vi "TwoSensorMagazineLogic.vi"(0 "Intake Toggle":bool, 1 "Outtake Button":bool, 2 "error in (no error)":errorcluster, 3 "Outtake Side Sensor":bool, 4 "Intake Side Sensor":bool) -> (5 "Current State":T1, 6 "Intake Pistons":bool, 7 "Magazine Motors":dbl, 8 "Kicker Motors":dbl, 9 "Intake Motors":dbl, 10 "error out":errorcluster)   [LabVIEW 2020]
uses:
  MagazineControl.ctl
  TitanLib/Lib/TitanLib.lvlib
panel:
  in  "Kicker Power":dbl=0.5
  in  "Magazine Power":dbl=1.0
  in  "Input Power":dbl=1.0
  in  "Initial State":T1
  # "Inputs"
  # "Power Levels"
  # "Outputs"
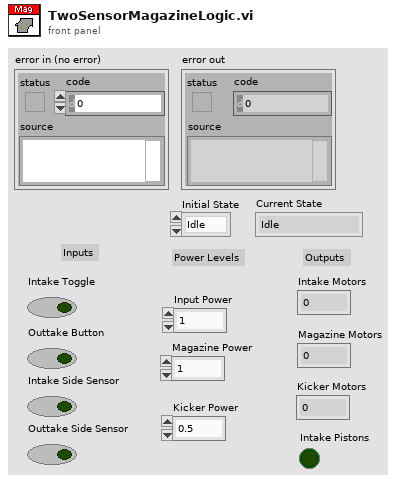
[diagram p1: front panel]
types:
  T1 = typedef "MagazineControl.ctl" = enum16{"Idle", "Intaking", "Outtake", "One Ball", "One Ball Intake", "One Ball Outtake", "Two Balls", "Two Ball Outtake"}
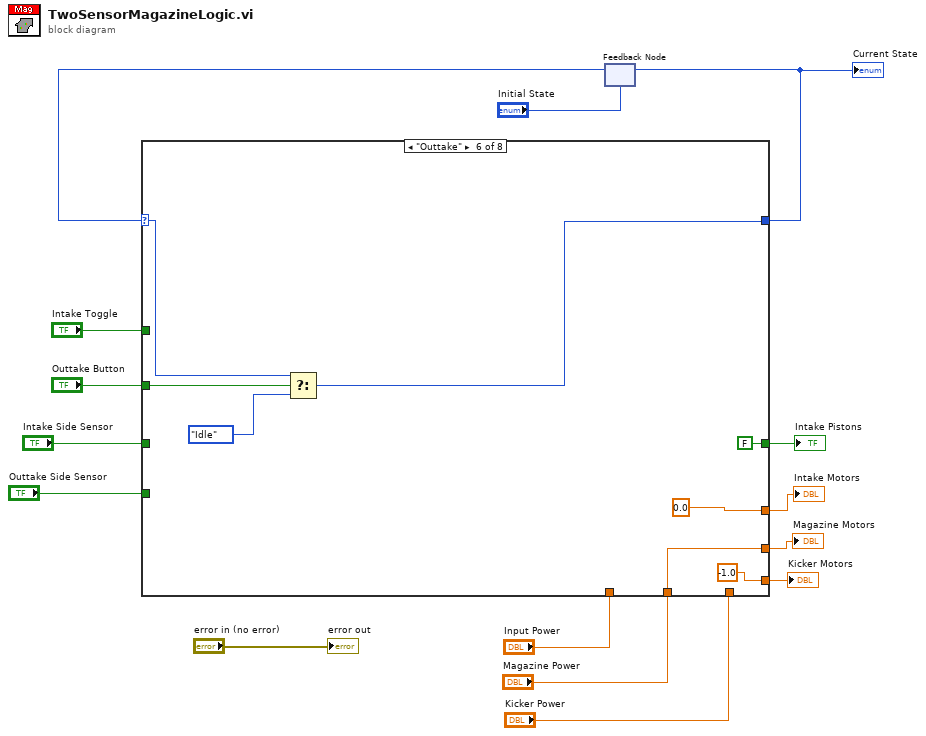
[diagram p0: block diagram]
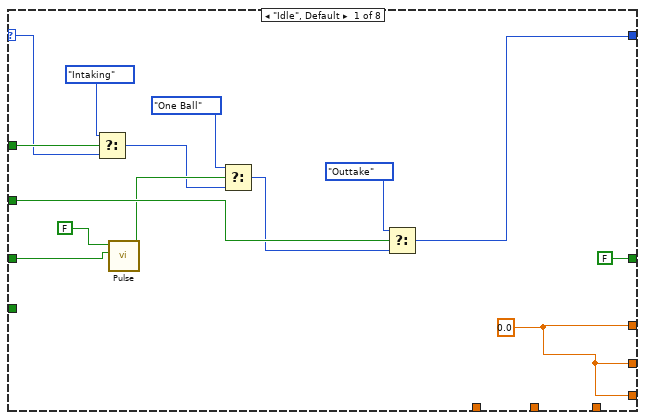
[diagram p2: hidden frame]
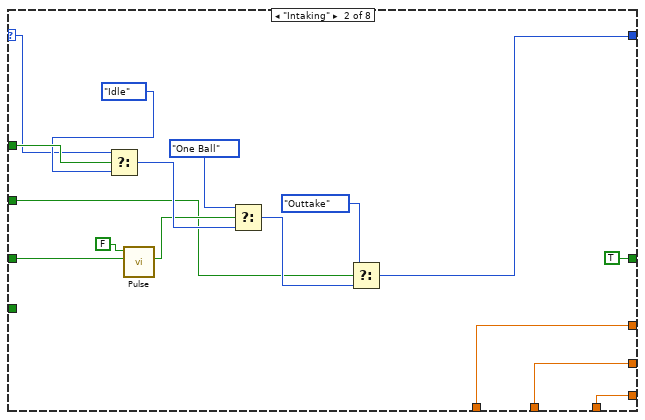
[diagram p3: hidden frame]
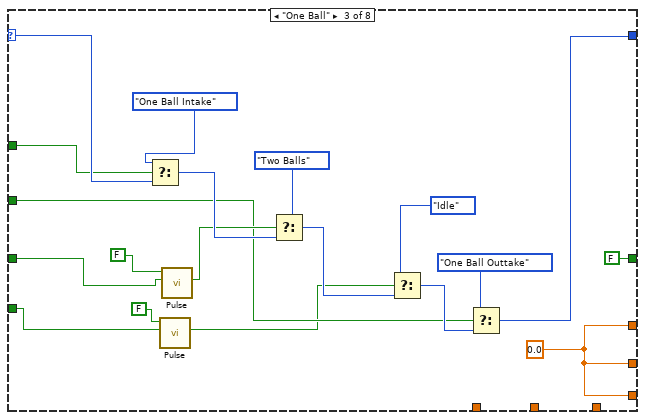
[diagram p4: hidden frame]
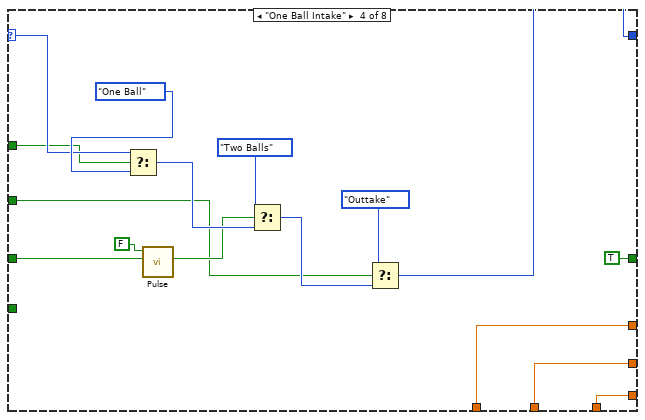
[diagram p5: hidden frame]
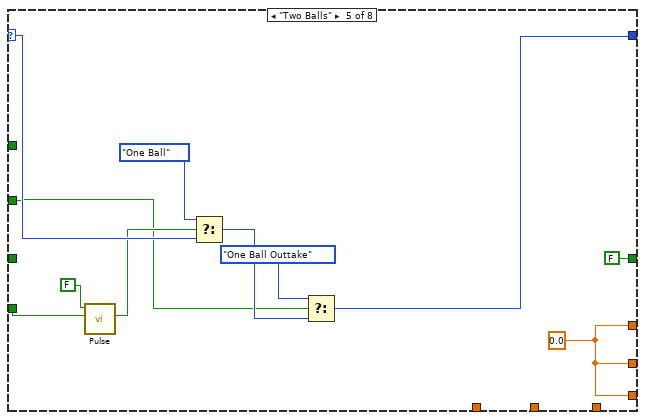
[diagram p6: hidden frame]
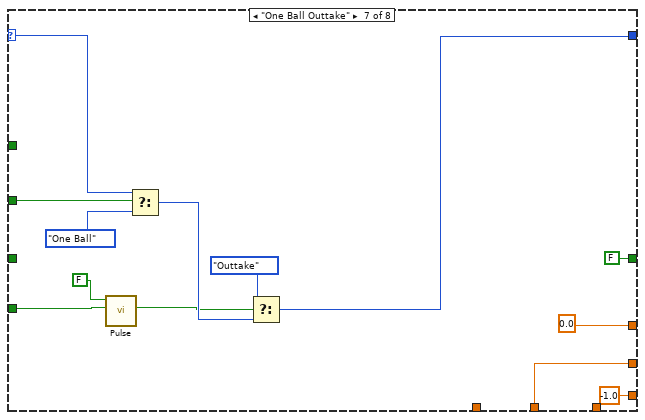
[diagram p7: hidden frame]
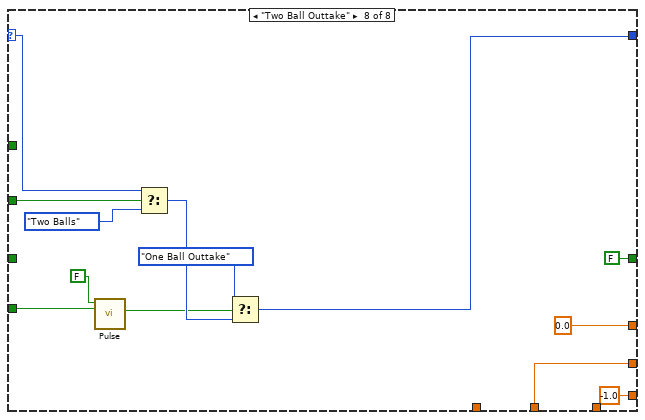
[diagram p8: hidden frame]
diagram:
  n1 = feedback #1("Initial State") -> (w4:T1)
  n2 = case shown="\"Outtake\"" w4 {
    selector: w4 -> [w27 w38 w57 w72 w91 w98 w108 w121]
    tunnel: "Intake Toggle" -> [w29 w40 w56 w71 _ _ _ _]
    tunnel: "Outtake Button" -> [w28 w30 w47 w65 w81 w99 w109 w122]
    tunnel: "Intake Side Sensor" -> [w22 w35 w58 w73 _ _ _ _]
    tunnel: [w16 w41 w52 w74 w88 w96 w104 w117] -> w3
    tunnel: [w20 w37 w55 w70 w89 0.0 ("Input Power") 0.0 ("Input Power") 0.0 ("Input Power")] -> w10
    tunnel: "Input Power" -> [_ w37 _ w70 _ _ _ _]
    tunnel: [w20 w36 w55 w69 w89 w93 w112 w125] -> w12
    tunnel: "Magazine Power" -> [_ w36 _ w69 _ w93 w112 w125]
    tunnel: [w20 w33 w55 w68 w89 -1.0 ("Kicker Motors") -1.0 ("Kicker Motors") -1.0 ("Kicker Motors")] -> w14
    tunnel: "Kicker Power" -> [_ w33 _ w68 _ _ _ _]
    tunnel: "Outtake Side Sensor" -> [_ _ w50 _ w85 _ w102 w116]
    tunnel: [FALSE ("Intake Pistons") TRUE ("Intake Pistons") FALSE ("Intake Pistons") TRUE ("Intake Pistons") FALSE ("Intake Pistons") FALSE ("Intake Pistons") FALSE ("Intake Pistons") FALSE ("Intake Pistons")] -> w2
    frame "Idle", Default {
      w20 = 0.0 ("Input Power")
      n3 = Select(t=MagazineControl."Intaking", s=w29, f=w27) -> (s? t:f=w17:T1)
      n4 = call "Pulse.vi"("Input"=w22, "Rising Edge?"=FALSE) -> ("Output"=w23:bool)  [unwired: 9 in]
      n5 = Select(t=MagazineControl."One Ball", s=w23, f=w17) -> (s? t:f=w18:T1)
      n6 = Select(t=MagazineControl."Outtake", s=w28, f=w18) -> (s? t:f=w16:T1)
    }
    frame "Intaking" {
      n7 = Select(t=w38, s=w40, f=MagazineControl."Idle" ("t")) -> (s? t:f=w44:T1)
      n8 = call "Pulse.vi"("Input"=w35, "Rising Edge?"=FALSE) -> ("Output"=w31:bool)  [unwired: 9 in]
      n9 = Select(t=MagazineControl."One Ball", s=w31, f=w44) -> (s? t:f=w45:T1)
      n10 = Select(t=MagazineControl."Outtake", s=w30, f=w45) -> (s? t:f=w41:T1)
    }
    frame "One Ball" {
      w55 = 0.0 ("Input Power")
      n11 = Select(t=MagazineControl."One Ball Intake", s=w56, f=w57) -> (s? t:f=w63:T1)
      n12 = call "Pulse.vi"("Input"=w50, "Rising Edge?"=FALSE) -> ("Output"=w46:bool)  [unwired: 9 in]
      n13 = call "Pulse.vi"("Input"=w58, "Rising Edge?"=FALSE) -> ("Output"=w48:bool)  [unwired: 9 in]
      n14 = Select(t=MagazineControl."Two Balls", s=w48, f=w63) -> (s? t:f=w64:T1)
      n15 = Select(t=MagazineControl."Idle", s=w46, f=w64) -> (s? t:f=w54:T1)
      n16 = Select(t=MagazineControl."One Ball Outtake", s=w47, f=w54) -> (s? t:f=w52:T1)
    }
    frame "One Ball Intake" {
      n17 = Select(t=w72, s=w71, f=MagazineControl."One Ball" ("t")) -> (s? t:f=w79:T1)
      n18 = call "Pulse.vi"("Input"=w73, "Rising Edge?"=FALSE) -> ("Output"=w66:bool)  [unwired: 9 in]
      n19 = Select(t=MagazineControl."Two Balls", s=w66, f=w79) -> (s? t:f=w80:T1)
      n20 = Select(t=MagazineControl."Outtake", s=w65, f=w80) -> (s? t:f=w74:T1)
    }
    frame "Two Balls" {
      w89 = 0.0 ("Input Power")
      n21 = call "Pulse.vi"("Input"=w85, "Rising Edge?"=FALSE) -> ("Output"=w82:bool)  [unwired: 9 in]
      n22 = Select(t=MagazineControl."One Ball", s=w82, f=w91) -> (s? t:f=w87:T1)
      n23 = Select(t=MagazineControl."One Ball Outtake", s=w81, f=w87) -> (s? t:f=w88:T1)
    }
    frame "Outtake" {
      n24 = Select(t=w98, s=w99, f=MagazineControl."Idle") -> (s? t:f=w96:T1)
    }
    frame "One Ball Outtake" {
      n25 = call "Pulse.vi"("Input"=w102, "Rising Edge?"=FALSE) -> ("Output"=w103:bool)  [unwired: 9 in]
      n26 = Select(t=w108, s=w109, f=MagazineControl."One Ball") -> (s? t:f=w106:T1)
      n27 = Select(t=MagazineControl."Outtake", s=w103, f=w106) -> (s? t:f=w104:T1)
    }
    frame "Two Ball Outtake" {
      n28 = call "Pulse.vi"("Input"=w116, "Rising Edge?"=FALSE) -> ("Output"=w115:bool)  [unwired: 9 in]
      n29 = Select(t=w121, s=w122, f=MagazineControl."Two Balls") -> (s? t:f=w119:T1)
      n30 = Select(t=MagazineControl."One Ball Outtake", s=w115, f=w119) -> (s? t:f=w117:T1)
    }
  }
  "Intake Motors" <- w10
  "Magazine Motors" <- w12
  "Kicker Motors" <- w14
  "Current State" <- w3
  "Intake Pistons" <- w2
  n31 = feedback-in #1(w3) -> ()
  "error out" <- "error in (no error)"
